vi "test Scheduled Loopback.vi"(8 "error in":errorcluster, 11 "TestCase in":refnum<class "Octal Loopback.lvclass">) -> (0 "error out":errorcluster, 3 "TestCase out":refnum<class "Octal Loopback.lvclass">)   [LabVIEW 2020, in "Octal Loopback.lvclass"]
uses:
  Octal Loopback.lvclass
  C:/Program Files (x86)/National Instruments/LabVIEW 2020/vi.lib/NI/VeriStand Custom Device Testing Tools/VeriStandTestCase/VeriStandTestCase.lvclass
  <vilib>/numeric/Random Number (Range) U64.vi
  <vilib>/numeric/sub_Random U32.vi
  <vilib>/addons/_JKI Toolkits/VI Tester/TestCase.llb/TestCase.lvclass
  <vilib>/NI/VeriStand Custom Device Testing Tools/VeriStandTestUtilities/VeriStandTestUtilities.lvlib
  C:/Program Files (x86)/National Instruments/LabVIEW 2020/vi.lib/addons/_JKI Toolkits/VI Tester/TestCase.llb/TestCase.lvclass
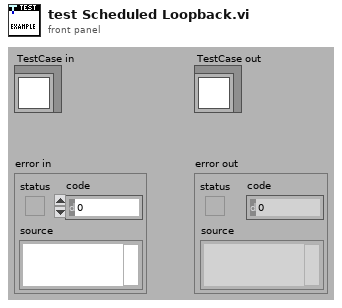
[diagram p1: front panel]
types:
  T1 = typedef "NI_VS Workspace ExecutionAPI.lvlib/WorkspaceAPI.ctl" = refnum<k24>
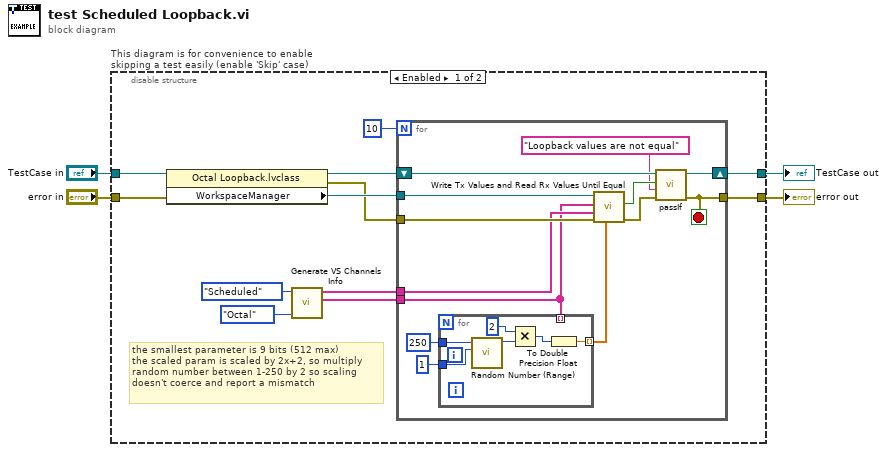
[diagram p0: block diagram]
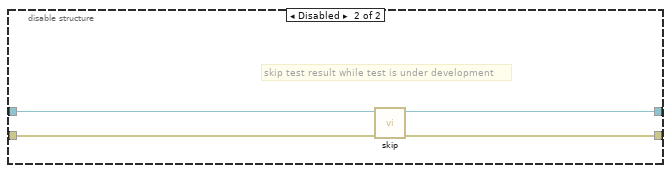
[diagram p2: hidden frame]
diagram:
  n1 = disable-structure "This diagram is for convenience to enable skipping a test easily (enable 'Skip' case)" shown="Enabled" {
    disable-tunnel: "TestCase in" -> [w11 w39]
    disable-tunnel: [w9 w37] -> w1
    disable-tunnel: [w8 w38] -> w3
    disable-tunnel: "error in" -> [w10 w36]
    frame Enabled {
      # "the smallest parameter is 9 bits (512 max)\nthe scaled param is scaled by 2x+2, so multiply \nrandom number between 1-250 by 2 so scaling\ndoesn't coerce and report a mismatch"
      n2 = property class="Octal Loopback.lvclass"(reference=w11, error in=w10) -> (reference out=w13:refnum<class "Octal Loopback.lvclass">, error out=w14:errorcluster, "WorkspaceManager"=w15:T1)
      n3 = call "Generate VS Channels Info.vi"("Label Format (Decimal)"=enum16{"Decimal", "Octal"}."Octal", "Transfer Type"=enum16{"Acyclic", "Scheduled"}."Scheduled") -> ("Tx Channels Array"=w7:string[], "Rx Channels Array"=w16:string[])  [unwired: 5 in, 3 out]
      n4 = for {
        N: 10 -> [_]
        tunnel: w16 -> [w18]
        tunnel: w15 -> [w29]
        tunnel: w14 -> [w28]
        tunnel: w7 -> [w17]
        shift-right: [w25] -> w9
        shift-left: w13 -> [w26]
        tunnel: [w24] -> w8
        stop <- w24 stop-if-true
        n5 = for {
          tunnel: [w34] -> w19 mode=indexing
          tunnel: u64 250 ("upper bound (100)") -> [w33]
          tunnel: u64 1 ("upper bound (100)") -> [w32]
          tunnel: w17 -> [_] mode=indexing
          n6 = call-poly <vilib>:"Random Number (Range).vi"("lower bound (0)"=w32, "upper bound (100)"=w33) -> ("number"=w35:u64)  [unwired: 9 in]
          n7 = Multiply(x=u64 2, y=w35) -> (x*y=w31:u64)
          n8 = To Double Precision Float(number=w31) -> (double precision float=w34:dbl)
        }
        n9 = call <vilib>:"Write Tx Values and Read Rx Values Until Equal.vi"("Tx values"=w19, "error in"=w28, "Rx aliases"=w18, "Tx aliases"=w17, "workspace manager in"=w29) -> ("error out"=w27:errorcluster, "values equal"=w23:bool)  [unwired: 4 in, 1 out]
        n10 = call-dynamic "passIf.vi"("error in (no error)"=w27, "message (\"\")"="Loopback values are not equal" ("message (\"\")"), "pass"=w23, "TestCase in"=w26) -> ("error out"=w24:errorcluster, "TestCase out"=w25:refnum<class "Octal Loopback.lvclass">)  [unwired: 6 in]
      }
    }
    frame Disabled {
      # "skip test result while test is under development"
      n11 = call <vilib>:"skip.vi"("error in (no error)"=w36, "TestCase in"=w39) -> ("error out"=w38:errorcluster, "TestCase out"=w37:refnum<class "Octal Loopback.lvclass">)  [unwired: 8 in]
    }
  }
  "error out" <- w3
  "TestCase out" <- w1
